vi "rqcBob Channel Test - 2 SPD (Low Level Example).vi"() -> ()   [LabVIEW 2018]
uses:
  FPGA/rqcBob/Custom Controls/Pulse Train/rqcBob Pulse Train Config.ctl
  FPGA/rqcBob/Custom Controls/Pulse Train/rqcBob Pulse Train.Generation Mode.ctl
  FPGA/rqcBob/Custom Controls/Pulse Train/rqcBob Pulse Train.First Pulse Delay Mode.ctl
  FPGA/rqcBob/Custom Controls/rqcBob Modulator Config.ctl
  FPGA/rqcBob/Custom Controls/rqcBob Window Config.ctl
  Shared/Shared FPGA Lib/Shared Logic/Custom Controls/rqc Random Generator.parameters.ctl
  Shared/Shared FPGA Lib/Shared Logic/Custom Controls/rqc Random Generator.value type.ctl
  FPGA/rqcBob/Custom Controls/rqcBob Trigger Type.ctl
  <vilib>/FPGAPlugInAG/PCIe-7820R/niLvFpga_Open_PCIe-7820R.vi
  <vilib>/rvi/interface/common/dynamic/niFpgaDynamicAddResources.vi
  Low Level API/Configuration/Photon Detector/Detection FIFOs config/rqcBob Configure PD Detect FIFO (2PD).vi
  Low Level API/Read/Read PD Detection FIFO/rqcBob Read PD Detection FIFO (1PD PD1).vi
  Low Level API/Read/Read PD Detection FIFO/rqcBob Read PD Detection FIFO (1PD PD2).vi
  <vilib>/FPGAPlugInAG/Dynamic/niLvFpga_Close_Dynamic.vi
  <vilib>/rvi/interface/nirviOpenFPGA/nirviOpenFPGA.xnode
  FPGA Bitfiles/rqcBob (FPGA) 7820 v 3.1.0.lvbitx
  <vilib>/rvi/interface/nirviCloseFPGA/nirviCloseFPGA.xnode
  <vilib>/Analysis/NI_AALBase.lvlib
panel:
  out "2-nd Detector Clicks":T1(graph)
  in  "modulator.clock delay":fxp<+,4,4>
  out "Done":bool=TRUE
  in  "train.software trigger":bool
  in  "stop":bool
  out "1-st Detector Clicks":T1(graph)
  in  "rndGen.parameters":T2={"value type"=enum."constant", "constant"=150, "num of levels"=4, "levels values"=[0, 0, 0, 0]}
  in  "window.config":T4={"window.open"=0, "window.close"=3000}
  in  "modulator.config":T5={"modulator.start"=1000, "modulator.stop"=2700}
  out "SPD.max meas length":u32=32000
  in  "train.configuration":T6={"period"=4000, "num of pulses"=1, "mode"=enum."train sequence.single", "num of trains"=4000, "first pulse delay mode"=enum."every train", "first pulse delay"=55}
  # "Bob configuration"
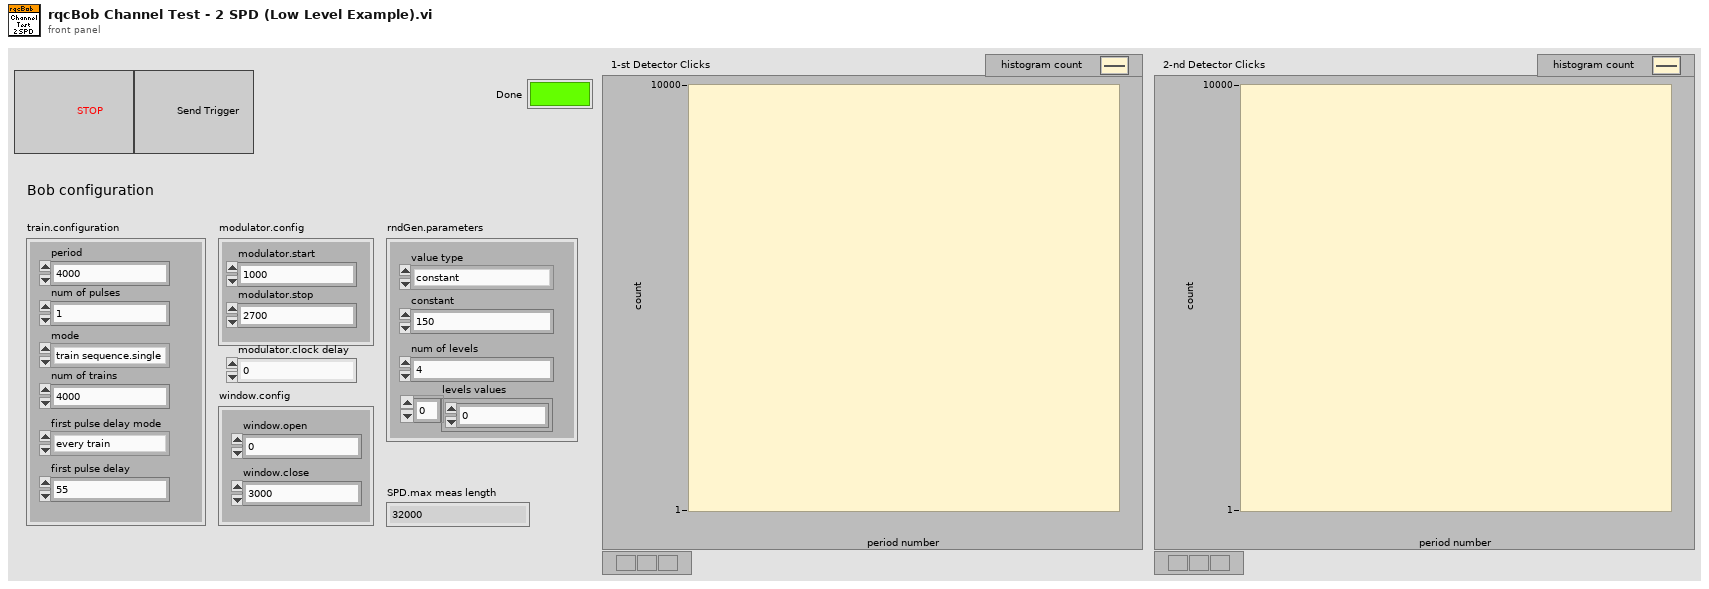
[diagram p1: front panel]
types:
  T1 = cluster{"X Values":dbl[], "Histogram: h(x)":i32[]}
  T2 = typedef "rqc Random Generator.parameters.ctl" = cluster{"value type":T3, "constant":u16, "num of levels":u16, "levels values":u16[]}
  T3 = typedef "rqc Random Generator.value type.ctl" = enum16{"random value", "constant"}
  T4 = typedef "rqcBob Window Config.ctl" = cluster{"window.open":u16, "window.close":u16}
  T5 = typedef "rqcBob Modulator Config.ctl" = cluster{"modulator.start":u16, "modulator.stop":u16}
  T6 = typedef "rqcBob Pulse Train Config.ctl" = cluster{"period":u16, "num of pulses":u16, "mode":T7, "num of trains":u16, "first pulse delay mode":T8, "first pulse delay":u16}
  T7 = typedef "rqcBob Pulse Train.Generation Mode.ctl" = enum8{"single train", "train sequence.single", "train sequence.wait for trigger", "continuous"}
  T8 = typedef "rqcBob Pulse Train.First Pulse Delay Mode.ctl" = enum8{"none", "every train", "first train"}
  T9 = typedef "rqcBob Trigger Type.ctl" = enum16{"software", "immediate", "DIO"}
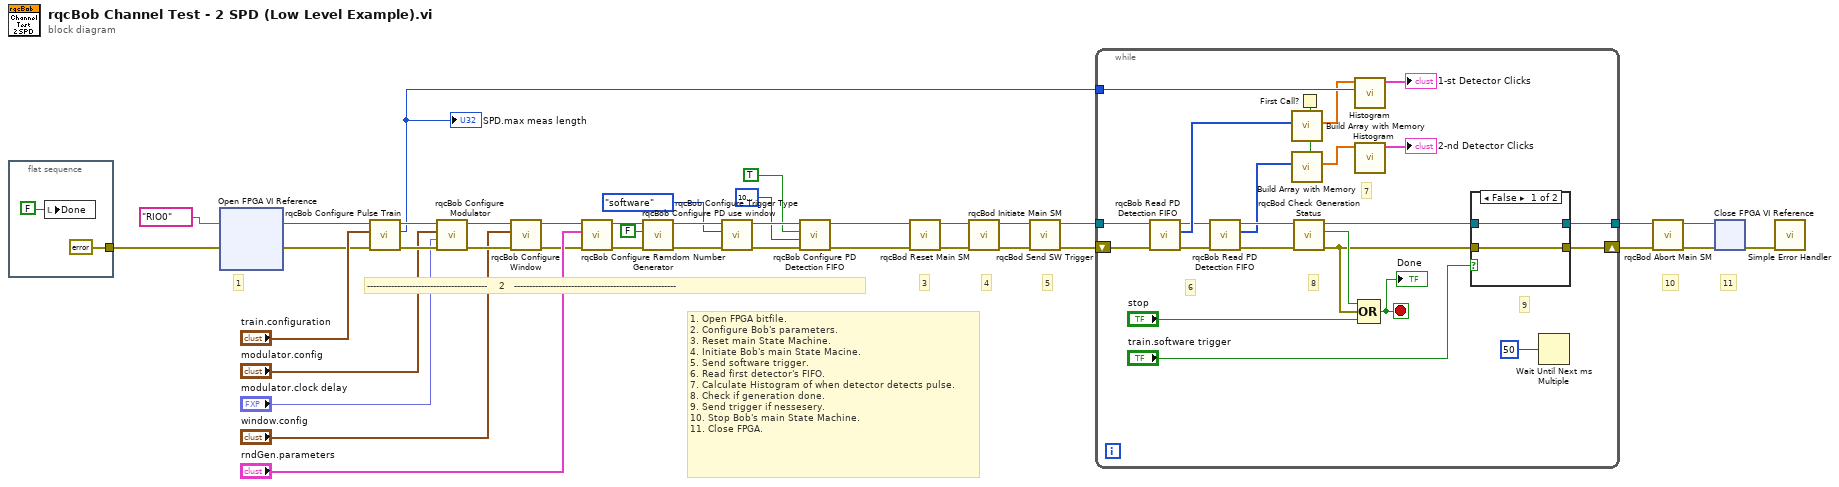
[diagram p0: block diagram]
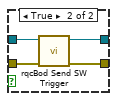
[diagram p2: hidden frame]
diagram:
  # "1. Open FPGA bitfile.\n2. Configure Bob's parameters.\n3. Reset main State Machine.\n4. Initiate Bob's main State Macine.\n5. Send software trigger.\n6. Read first detector's FIFO.\n7. Calculate Histogram of when detector detects pulse.\n8. Check if generation done.\n9. Send trigger if nessesery.\n10. Stop Bob's main State Machine.\n11. Close FPGA."
  # "1"
  # "11"
  # "10"
  # "5"
  # "4"
  # "3"
  # "----------------------------------------    2   ------------------------------------------------------"
  n1 = flat-sequence {
    tunnel: [errorcluster {"status"=FALSE, "code"=0, "source"=""} ("error in")] -> w13
    frame #0 {
      n2 = local write "Done"(FALSE ("Done")) -> ()
    }
  }
  n3 = xnode "Open FPGA VI Reference"("error in"=w13, "resource name"=tag "RIO0") -> ("FPGA VI Reference Out"=w10:refnum<k20>, "error out"=w9:errorcluster)
  n4 = call "rqcBob Configure Pulse Train.vi"("error in"=w9, "train.configuration"="train.configuration", "FPGA reference in"=w10) -> ("error out"=w36:errorcluster, "SPD meas length"=w17:u32, "FPGA reference out"=w37:refnum<k20>)  [unwired: 6 in]
  "SPD.max meas length" <- w17
  n5 = call "rqcBob Configure Modulator.vi"("error in"=w36, "modulator.clock delay"="modulator.clock delay", "modulator.config"="modulator.config", "FPGA reference in"=w37) -> ("error out"=w33:errorcluster, "FPGA reference out"=w34:refnum<k20>)  [unwired: 6 in]
  n6 = call "rqcBob Configure Window.vi"("error in"=w33, "window.config"="window.config", "FPGA reference in"=w34) -> ("error out"=w29:errorcluster, "FPGA reference out"=w30:refnum<k20>)  [unwired: 7 in]
  n7 = call "rqcBob Configure Ramdom Number Generator.vi"("error in"=w29, "rqcBob rndGen.parameters"="rndGen.parameters", "FPGA reference in"=w30) -> ("error out"=w28:errorcluster, "FPGA reference out"=w27:refnum<k20>)  [unwired: 7 in]
  n8 = call "rqcBob Configure PD use window.vi"("error in"=w28, "PD.use window"=FALSE ("SPD.use detector window"), "FPGA reference in"=w27) -> ("error out"=w25:errorcluster, "FPGA reference out"=w26:refnum<k20>)  [unwired: 7 in]
  n9 = call "rqcBob Configure Trigger Type.vi"("error in"=w25, "rqcBob Trigger Type"=rqcBob_Trigger_Type."software", "FPGA reference in"=w26) -> ("error out"=w5:errorcluster, "FPGA reference out"=w7:refnum<k20>)  [unwired: 7 in]
  n10 = call-poly "rqcBob Configure PD Detection FIFO.vi"("error in"=w5, "PD.detect fifo depth"=u32 1000000 ("SPD.detect fifo depth"), "PD.detect fifo write enable"=TRUE ("SPD.detect fifo write enable"), "FPGA reference in"=w7) -> ("error out"=w4:errorcluster, "FPGA reference out"=w6:refnum<k20>)  [unwired: 6 in]
  n11 = call "rqcBod Reset Main SM.vi"("error in"=w4, "FPGA reference in"=w6) -> ("error out"=w22:errorcluster, "FPGA reference out"=w23:refnum<k20>)  [unwired: 8 in]
  n12 = call "rqcBod Initiate Main SM.vi"("error in"=w22, "FPGA reference in"=w23) -> ("error out"=w20:errorcluster, "FPGA reference out"=w21:refnum<k20>)  [unwired: 8 in]
  n13 = call "rqcBod Send SW Trigger.vi"("error in"=w20, "FPGA reference in"=w21) -> ("error out"=w18:errorcluster, "FPGA reference out"=w19:refnum<k20>)  [unwired: 8 in]
  n14 = while {
    tunnel: w19 -> [w54]
    shift-right: [w59] -> w16
    shift-left: w18 -> [w52]
    tunnel: w17 -> [w62]
    tunnel: [w58] -> w1
    stop <- w56 stop-if-true
    # "7"
    # "9"
    # "8"
    # "6"
    n15 = call-poly "rqcBob Read PD Detection FIFO.vi"("error in"=w52, "FPGA reference in"=w54) -> ("error out"=w44:errorcluster, "Data"=w53:u32[], "FPGA reference out"=w46:refnum<k20>)  [unwired: 6 in, 1 out]
    n16 = call-poly "rqcBob Read PD Detection FIFO.vi"("error in"=w44, "FPGA reference in"=w46) -> ("error out"=w43:errorcluster, "Data"=w42:u32[], "FPGA reference out"=w45:refnum<k20>)  [unwired: 6 in, 1 out]
    n17 = call "rqcBod Check Generation Status.vi"("error in"=w43, "FPGA reference in"=w45) -> ("error out"=w60:errorcluster, "generation.done"=w63:bool, "FPGA reference out"=w61:refnum<k20>)  [unwired: 7 in]
    n18 = First Call?() -> (First Call?: T/F=w49:bool)
    n19 = call "Build Array with Memory.vi"("reset"=w49, "new array"=w53) -> ("appended array"=w51:dbl[])  [unwired: 9 in]
    n20 = call "Build Array with Memory.vi"("reset"=w49, "new array"=w42) -> ("appended array"=w47:dbl[])  [unwired: 9 in]
    n21 = call <vilib>:"Histogram.vi"("intervals"=w62, "X"=w51) -> ("Histogram Graph"=→"1-st Detector Clicks":T1)  [unwired: 6 in, 3 out]
    n22 = call <vilib>:"Histogram.vi"("X"=w47) -> ("Histogram Graph"=→"2-nd Detector Clicks":T1)  [unwired: 7 in, 3 out]
    n23 = Compound Arithmetic op=OR(w63, w60, "stop") -> (w56:bool)
    "Done" <- w56
    n24 = case shown="False" "train.software trigger" {
      tunnel: w61 -> [w66 w70]
      tunnel: w60 -> [w65 w69]
      tunnel: [w66 w68] -> w58
      tunnel: [w65 w67] -> w59
      frame False {
      }
      frame True {
        n25 = call "rqcBod Send SW Trigger.vi"("error in"=w69, "FPGA reference in"=w70) -> ("error out"=w67:errorcluster, "FPGA reference out"=w68:refnum<k20>)  [unwired: 8 in]
      }
    }
    n26 = Wait Until Next ms Multiple(millisecond multiple=u32 50) -> ()  [unwired: 1 out]
  }
  n27 = call "rqcBod Abort Main SM.vi"("error in"=w16, "FPGA reference in"=w1) -> ("error out"=w14:errorcluster, "FPGA reference out"=w15:refnum<k20>)  [unwired: 8 in]
  n28 = xnode "Close FPGA VI Reference"("FPGA VI Reference In"=w15, "error in"=w14) -> ("error out"=w12:errorcluster)
  n29 = call <vilib>:"Simple Error Handler.vi"("error in (no error)"=w12) -> ()  [unwired: 4 in, 5 out]
